vi "Send Command.vi"(8 "error in (no error)":errorcluster, 9 "Delay Time (s)":dbl=1.0, 10 "Functions Control":T1, 11 "VISA resource name":refnum<visa-resource-name>) -> (0 "error out":errorcluster, 3 "VISA resource name out":refnum<visa-resource-name>)   [LabVIEW 2025]
uses:
  Functions Control.ctl
panel:
  out "read return count":u32
  out "read buffer":string
  out "write return count":u32
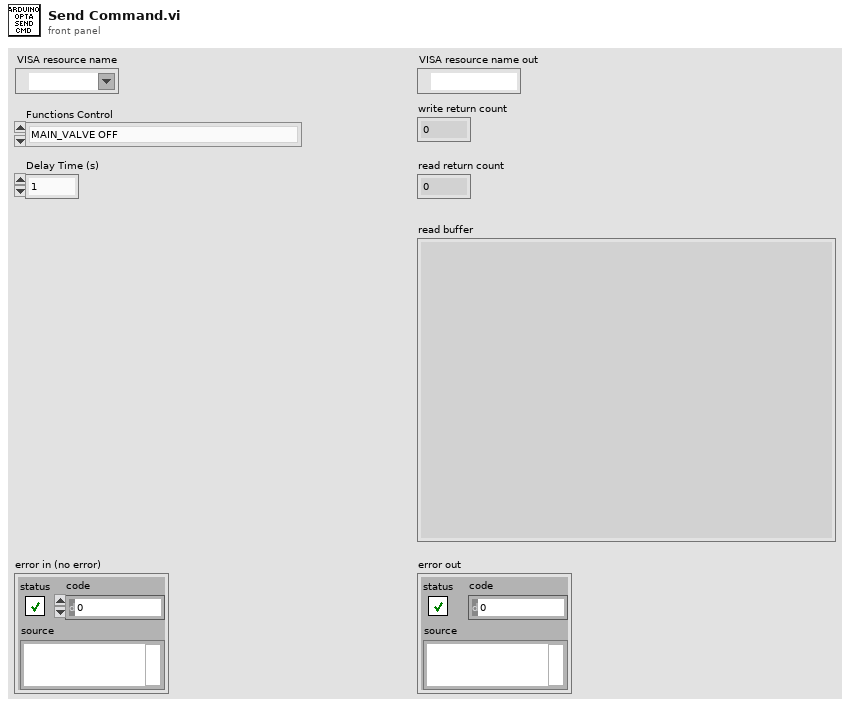
[diagram p1: front panel]
types:
  T1 = typedef "Functions Control.ctl" = enum16{"MAIN_VALVE OFF", "MAIN_VALVE ON", "VALVE1 OFF", "VALVE1 ON", "VALVE2 OFF", "VALVE2 ON", "VALVE3 OFF", "VALVE3 ON", "VALVE4 OFF", "VALVE4 ON", "VALVE5 OFF", "VALVE5 ON", "VALVE6 OFF", "VALVE6 ON", "FIX_POWER OFF", "FIX_POWER ON", "SPARE1 OFF", "SPARE1 ON", "SPARE2 OFF", "SPARE2 ON", "SPARE3 OFF", "SPARE3 ON", "SPARE4 OFF", "SPARE4 ON", "SPARE5 OFF", "SPARE5 ON", "RESET", "QUERY STATUS"}
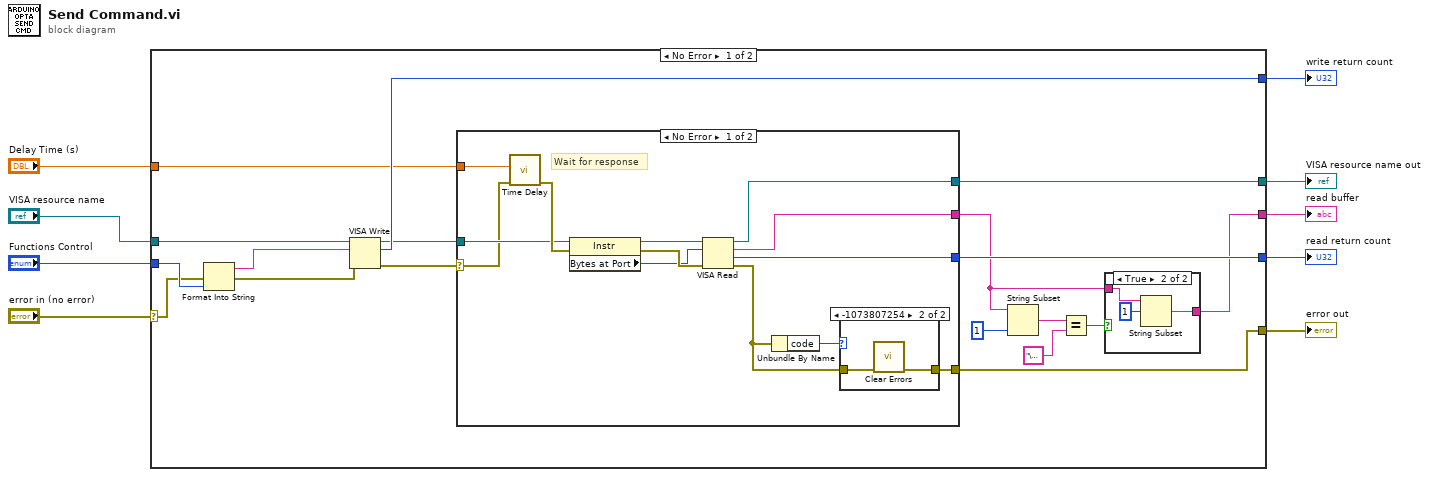
[diagram p0: block diagram]
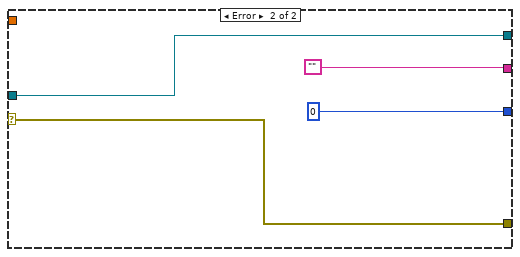
[diagram p4: hidden frame]
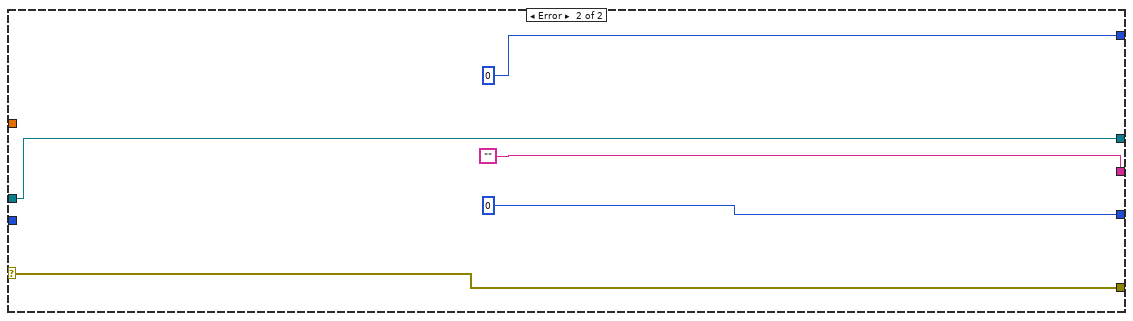
[diagram p5: hidden frame]
diagram:
  n1 = case shown="No Error" "error in (no error)" {
    selector: "error in (no error)" -> [w11 w53]
    tunnel: "VISA resource name" -> [w20 w56]
    tunnel: [w27 u32 0 ("return count")] -> w8
    tunnel: "Delay Time (s)" -> [w26 _]
    tunnel: [w24 w56] -> w6
    tunnel: [w23 w53] -> w5
    tunnel: [w18 ""] -> w4
    tunnel: [w22 u32 0 ("return count")] -> w3
    tunnel: "Functions Control" -> [w13 _]
    frame No Error {
      n2 = Format Into String(error in=w11, w13) -> (resulting string=w12:string, error out=w10:errorcluster)  [unwired: 2 in]
      n3 = VISA Write(VISA resource name=w20, write buffer=w12, error in (no error)=w10) -> (VISA resource name out=w25:refnum<visa-resource-name>, return count=w27:u32, error out=w21:errorcluster)
      n4 = case shown="No Error" w21 {
        selector: w21 -> [w35 w50]
        tunnel: w26 -> [w44 _]
        tunnel: w25 -> [w42 w51]
        tunnel: [w38 w51] -> w24
        tunnel: [w34 w50] -> w23
        tunnel: [w37 ""] -> w19
        tunnel: [w36 u32 0 ("return count")] -> w22
        frame No Error {
          # "Wait for response"
          n5 = call "Time Delay"("error in (no error)"=w35, "Delay Time (s)"=w44) -> ("error out"=w43:errorcluster)  [unwired: 9 in]
          n6 = property class="Instr"(reference=w42, error in=w43) -> (reference out=w41:refnum<visa-resource-name>, error out=w40:errorcluster, "Bytes at Port"=w39:u32)
          n7 = VISA Read(VISA resource name=w41, byte count=w39, error in (no error)=w40) -> (VISA resource name out=w38:refnum<visa-resource-name>, read buffer=w37:string, return count=w36:u32, error out=w33:errorcluster)
          n8 = Unbundle By Name(w33) -> ("code"=w32:i32)
          n9 = case shown="-1073807254" w32 {
            tunnel: w33 -> [w45 w47]
            tunnel: [w45 w46] -> w34
            frame Default {
            }
            frame -1073807254 {
              n10 = call <vilib>:"Clear Errors.vi"("error in (no error)"=w47) -> ("error out"=w46:errorcluster)  [unwired: 5 in, 1 out]
            }
          }
        }
        frame Error {
        }
      }
      n11 = String Subset(string=w19, length (rest)=1 ("offset (0)")) -> (substring=w17:string)  [unwired: 1 in]
      n12 = Equal?(x=w17, y="\u0000") -> (x = y?=w14:bool)
      n13 = case shown="True" w14 {
        tunnel: w19 -> [w28 w31]
        tunnel: [w28 w29] -> w18
        frame False {
        }
        frame True {
          n14 = String Subset(string=w31, offset (0)=1) -> (substring=w29:string)  [unwired: 1 in]
        }
      }
    }
    frame Error {
    }
  }
  "error out" <- w5
  "VISA resource name out" <- w6
  "write return count" <- w8
  "read buffer" <- w4
  "read return count" <- w3
